vi "Handle System Error.vi"(7 "Interactive?":bool=TRUE, 10 "error to handle":errorcluster, 11 "Mag Lab Error Handler in":refnum<class "Mag Lab Error Handler.lvclass">) -> (3 "Mag Lab Error Handler out":refnum<class "Mag Lab Error Handler.lvclass">)   [LabVIEW 2015, in "Mag Lab Error Handler.lvlib" / "Mag Lab Error Handler.lvclass"]
uses:
  Mag Lab Error Handler.lvclass
  <vilib>/Utility/error.llb/DialogType.ctl
  <vilib>/ActorFramework/Actor/Actor.lvclass/Actor.ctl
  Mag Lab Measure Controller Messages/Log Status Update Msg/Log Status Update Msg.lvclass/Log Status Update Msg.ctl
  <vilib>/ActorFramework/Message Enqueuer/Message Enqueuer.lvclass/Message Enqueuer.ctl
  Mag Lab Error Handler.lvclass/Mag Lab Error Handler.ctl
  <vilib>/ActorFramework/Stop Msg/Stop Msg.lvclass/Stop Msg.ctl
  <vilib>/ActorFramework/Message Enqueuer/Enqueue.vi
  <vilib>/ActorFramework/Stop Msg/Send Emergency Stop.vi
  <vilib>/ActorFramework/Message Enqueuer/Enqueue Critical.vi
  <vilib>/ActorFramework/Message Priority Queue/Priority Enqueue.vi
  Mag Lab Measure Controller Messages/Log Status Update Msg/Log Status Update Msg.lvclass
  <vilib>/ActorFramework/Stop Msg/Stop Msg.lvclass
  <vilib>/ActorFramework/Actor/Actor.lvclass
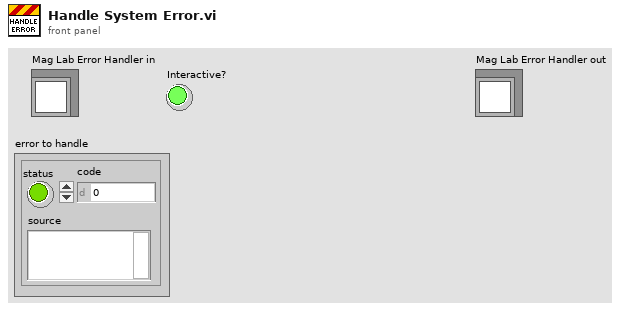
[diagram p1: front panel]
types:
  T1 = typedef "DialogType.ctl" = u16
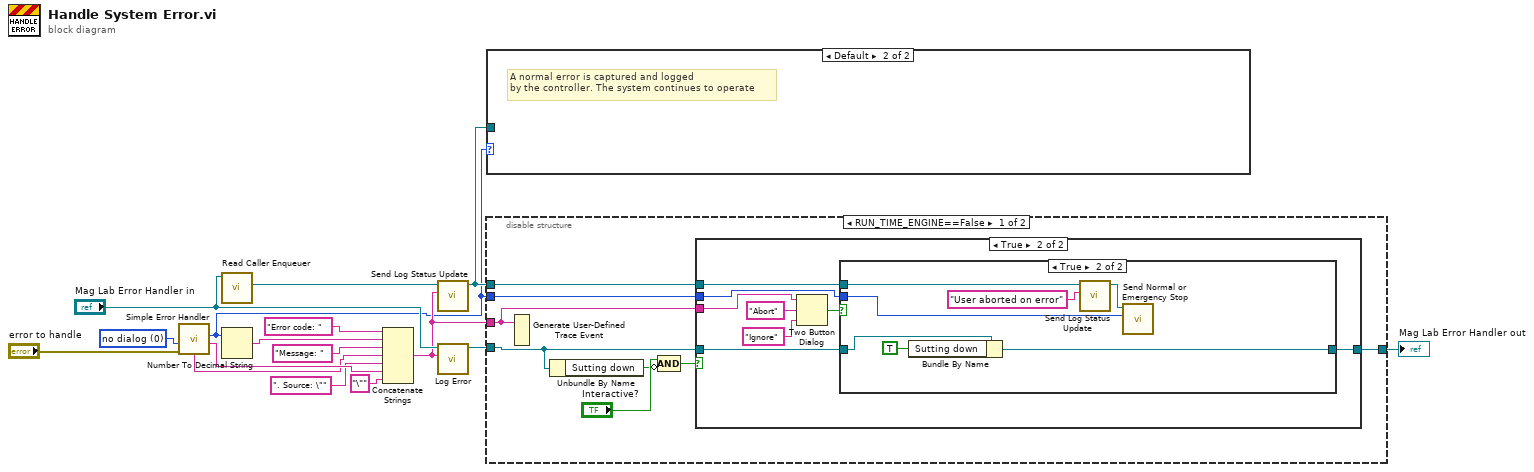
[diagram p0: block diagram]
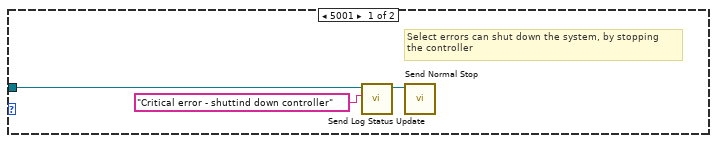
[diagram p2: hidden frame]
diagram:
  w7 = T1 0 items=["no dialog", "OK message", "continue or stop message", "OK message + warnings", "continue/stop + warnings"] ("type of dialog (OK msg:1)")
  n1 = call <vilib>:"Simple Error Handler.vi"("type of dialog (OK msg:1)"=w7, "error in (no error)"="error to handle") -> ("code out"=w4:i32, "source out"=w5:string, "message"=w2:string)  [unwired: 3 in, 2 out]
  n2 = call <vilib>:"Read Caller Enqueuer.vi"("Actor"="Mag Lab Error Handler in") -> ("Caller Enqueuer"=w13:refnum<class "Message Enqueuer.lvclass">)  [unwired: 10 in]
  n3 = Number To Decimal String(number=w4) -> (decimal integer string=w16:string)  [unwired: 1 in]
  n4 = Concatenate Strings("Error code: " ("string"), w16, "Message: " ("string"), w2, ". Source: \"" ("string"), w5, "\"" ("string")) -> (w8:string)
  n5 = call "Send Log Status Update.vi"("Status"=w8, "Message Enqueuer"=w13) -> ("Message Enqueuer out"=w12:refnum<class "Message Enqueuer.lvclass">)  [unwired: 8 in, 1 out]
  n6 = call "Log Error.vi"("Error"=w8, "Mag Lab Error Handler in"="Mag Lab Error Handler in") -> ("Mag Lab Error Handler out"=w9:refnum<class "Mag Lab Error Handler.lvclass">)  [unwired: 8 in, 1 out]
  n7 = case shown="Default" w4 {
    tunnel: w12 -> [w18 _]
    frame 5001 {
      # "Select errors can shut down the system, by stopping\nthe controller"
      n8 = call "Send Log Status Update.vi"("Status"="Critical error - shuttind down controller" ("String"), "Message Enqueuer"=w18) -> ("Message Enqueuer out"=w17:refnum<class "Message Enqueuer.lvclass">)  [unwired: 8 in, 1 out]
      n9 = call <vilib>:"Send Normal Stop.vi"("Message Enqueuer"=w17) -> ()  [unwired: 10 in, 1 out]
    }
    frame Default {
      # "A normal error is captured and logged\nby the controller. The system continues to operate"
    }
  }
  n10 = disable-structure shown="RUN_TIME_ENGINE==False" {
    disable-tunnel: w8 -> [w27 _]
    disable-tunnel: w12 -> [w25 _]
    disable-tunnel: w4 -> [w24 _]
    disable-tunnel: w9 -> [w22 _]
    disable-tunnel: [w23 _] -> w11
    frame condition #0 (active) {
      n11 = Generate User-Defined Trace Event(2:w27) -> ()  [unwired: 1 in]
      n12 = Unbundle By Name(w22) -> ("Sutting down"=w20:bool)
      n13 = Compound Arithmetic op=AND("Interactive?", invert w20) -> (w21:bool)
      n14 = case shown="True" w21 {
        tunnel: w27 -> [_ w36]
        tunnel: w25 -> [_ w33]
        tunnel: w24 -> [_ w31]
        tunnel: w22 -> [w28 w30]
        tunnel: [w28 w29] -> w23
        frame False {
        }
        frame True {
          n15 = Two Button Dialog(message=w36, 1:"Ignore" ("F button name (\"Cancel\")"), 2:"Abort" ("F button name (\"Cancel\")")) -> (T button?=w32:bool)
          n16 = case shown="True" w32 {
            tunnel: w33 -> [_ w43]
            tunnel: w31 -> [_ w41]
            tunnel: w30 -> [w37 w40]
            tunnel: [w37 w38] -> w29
            frame False {
            }
            frame True {
              n17 = Bundle By Name(cluster=w40, "Sutting down"=TRUE) -> (w38:refnum<class "Mag Lab Error Handler.lvclass">)
              n18 = call "Send Log Status Update.vi"("Status"="User aborted on error", "Message Enqueuer"=w43) -> ("Message Enqueuer out"=w44:refnum<class "Message Enqueuer.lvclass">)  [unwired: 8 in, 1 out]
              n19 = call <vilib>:"Send Normal or Emergency Stop.vi"("final error code"=w41, "Message Enqueuer"=w44) -> ()  [unwired: 9 in, 1 out]
            }
          }
        }
      }
    }
    frame condition #1 {
    }
  }
  "Mag Lab Error Handler out" <- w11
